vi "SoundInput-DAQ.vi"(7 "Name(\"\" to use uuid)":string="Acquisition") -> ()   [LabVIEW 2017, in "SoundInput-DAQ.lvlib"]
uses:
  SoundInput-DAQ.lvlib
  <vilib>/sound2/lvsound2.llb/Sound Data Format.ctl
  <vilib>/sound2/lvsound2.llb/Sampling Mode.ctl
  bc6f9ce3-7135-4df3-9fce-67397201bd09.vi
  f3e3012a-dc83-45d7-82c5-490bef76f43f.vi
  e2413101-be31-4c43-921b-7e7496268bc5.vi
  07cbb487-6694-43fd-ac53-f2be3466fcff.vi
  fecb174d-6823-407c-a974-ffebb4610b14.vi
  0bf643a1-791c-4b4c-b91f-da80b9c7e2fb.vi
  041ba748-83ae-40d3-86c4-8e2f4b565384.vi
  <userlib>/_NEVSTOP/Communicable State Machine(CSM)/AdvanceAPI/CSM - Revert Arguments-Safe String.vi
  <userlib>/_NEVSTOP/Communicable State Machine(CSM)/_Shared/Trim Single-line Text.vi
  <userlib>/_NEVSTOP/Communicable State Machine(CSM)/AdvanceAPI/CSM - Make String Arguments Safe.vi
  <userlib>/_NEVSTOP/Communicable State Machine(CSM)/AdvanceAPI/CSM - Break Down Multiple States String.vi
  <userlib>/_NEVSTOP/Communicable State Machine(CSM)/AdvanceAPI/CSM - Compact Multiple States.vi
  f3e3012a-dc83-45d7-82c5-490bef76f43f.vi/99de0c97-112a-4c86-9094-c187659127e1.vi
  <userlib>/_NEVSTOP/Communicable State Machine(CSM)/Utility/Build Error Cluster.vi
  0bf643a1-791c-4b4c-b91f-da80b9c7e2fb.vi/99de0c97-112a-4c86-9094-c187659127e1.vi
  <userlib>/_NEVSTOP/Communicable State Machine(CSM)/AdvanceAPI/CSM - Keywords.vi
  <vilib>/Utility/Data Type/Get Type Information.vi
  <userlib>/_NEVSTOP/Communicable State Machine(CSM)/addons/API-String-Arugments-Support/_Support/Data To SingleElementsArray_csm.vi
  <userlib>/_NEVSTOP/Communicable State Machine(CSM)/addons/API-String-Arugments-Support/_Support/Data To API String Arguments.vi
  <userlib>/_NEVSTOP/Communicable State Machine(CSM)/addons/INI-Static-Variable-Support/_Support/Parse Used Session and Name.vi
  <userlib>/_NEVSTOP/Communicable State Machine(CSM)/addons/INI-Static-Variable-Support/_Support/INI-FGV(lvlibp).vi
  <userlib>/_NEVSTOP/Communicable State Machine(CSM)/addons/INI-Static-Variable-Support/_Support/Populate String with INI Variable.vi
  <userlib>/_NEVSTOP/Communicable State Machine(CSM)/addons/API-String-Arugments-Support/_Support/Convert API String Arguments to Data(variant).vi
  <userlib>/_NEVSTOP/Communicable State Machine(CSM)/addons/API-String-Arugments-Support/_Support/SingleElementsArray To Data_csm.vi
  <userlib>/_NEVSTOP/Communicable State Machine(CSM)/addons/API-String-Arugments-Support/_Support/Query Data as API String Arguments(variant).vi
  <vilib>/sound2/lvsound2.llb/Sound Input Read (DBL).vi
  <userlib>/_NEVSTOP/Communicable State Machine(CSM)/addons/MassData-Parameter/_support/FGV-MassData(lvlibp).vi
  <userlib>/_NEVSTOP/Communicable State Machine(CSM)/_Polymophic/Add State(s) to Queue By BOOL(Element).vi
  <userlib>/_NEVSTOP/Communicable State Machine(CSM)/_Polymophic/CSM - Filter Duplicated Lines.vi
  <userlib>/_NEVSTOP/Communicable State Machine(CSM)/_Polymophic/CSM - Replace Marks in Messages.vi
  <userlib>/_NEVSTOP/Communicable State Machine(CSM)/Communicable State Machine.lvlib
  <userlib>/_NEVSTOP/Communicable State Machine(CSM)/addons/Loop-Support/CSM Loop Support.lvlib
  <userlib>/_NEVSTOP/Communicable State Machine(CSM)/_Shared/CSM Shared.lvlib
panel:
  in  "Sound Format":T1={"sample rate (S/s)"=20000.0, "number of channels"=2, "bits per sample"=16}
  in  "Device ID":u32 format="%.0x"
  in  "SamplePeroid(ms)":i32=200
  out "Raw Data":waveform(dbl)[](graph)
  in  "Cancel Button":bool
  in  "OK Button":bool
  out "Error Occurred":errorcluster
  out "State History":string
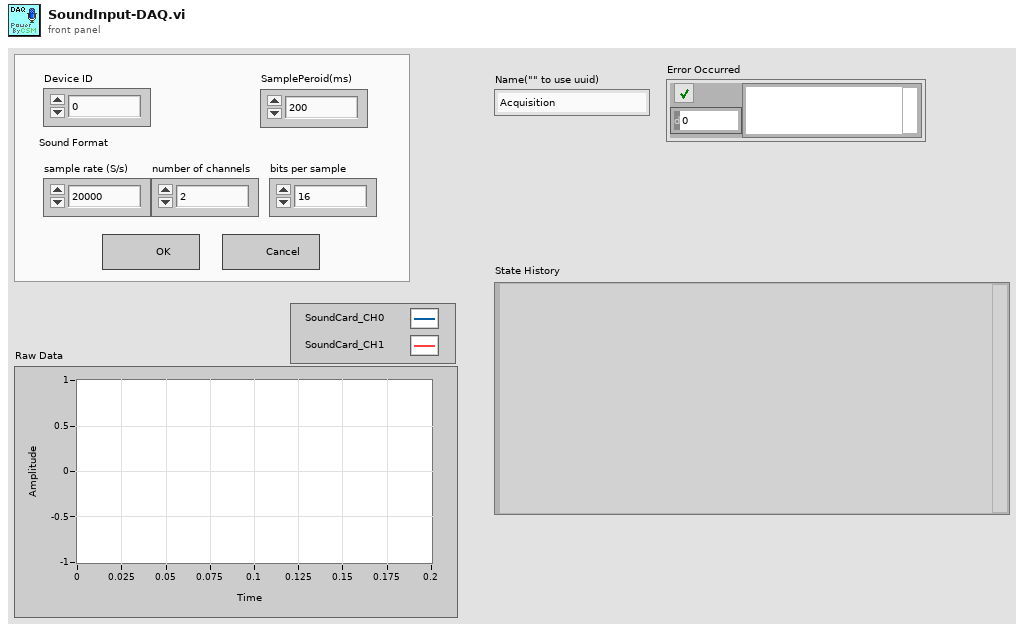
[diagram p1: front panel]
types:
  T1 = cluster{"sample rate (S/s)":dbl, "number of channels":i32, "bits per sample":i32}
  T2 = enum32{"Invalid", "Default", "Floating", "Floating/Auto-Hide", "Modal"}
  T3 = cluster{"Device ID":u32, "SamplePeroid(ms)":i32, "Sound Format":cluster{"sample rate (S/s)":dbl, "number of channels":i32, "bits per sample":i32}}
  T4 = enum32{"Invalid", "Standard", "Closed", "Hidden", "Minimized", "Maximized"}
  T5 = enum32{"invalid app kind", "Development System", "Run Time System", "Student Edition", "Embedded LabVIEW", "Evaluation", "Custom"}
  T6 = typedef "Communicable State Machine.lvlib/_CSM_Response Source Message.ctl" = cluster{"‘State":string, "’Arguments":string, "’Error":errorcluster}
  T7 = cluster{"Current VI Reference":refnum<vi>, "Close Panel on Exit?":bool}
  T8 = typedef "Sound Data Format.ctl" = cluster{"sample rate (S/s)":dbl, "number of channels":i32, "bits per sample":i32}
  T9 = cluster{"Core":cluster{"Current VI Reference":refnum<vi>, "Close Panel on Exit?":bool}, "Configuration":cluster{"Device ID":u32, "SamplePeroid(ms)":i32, "Sound Format":T8}, "State":enum16{"Idle", "Acquiring"}, "Number of Samples/ch":i32, "timestamp":timestamp}
  T10 = cluster{"Device ID":u32, "SamplePeroid(ms)":i32, "Sound Format":T8}
  T11 = typedef "Sampling Mode.ctl" = i32
  T12 = typedef "Sound Input Task ID.ctl" = u32
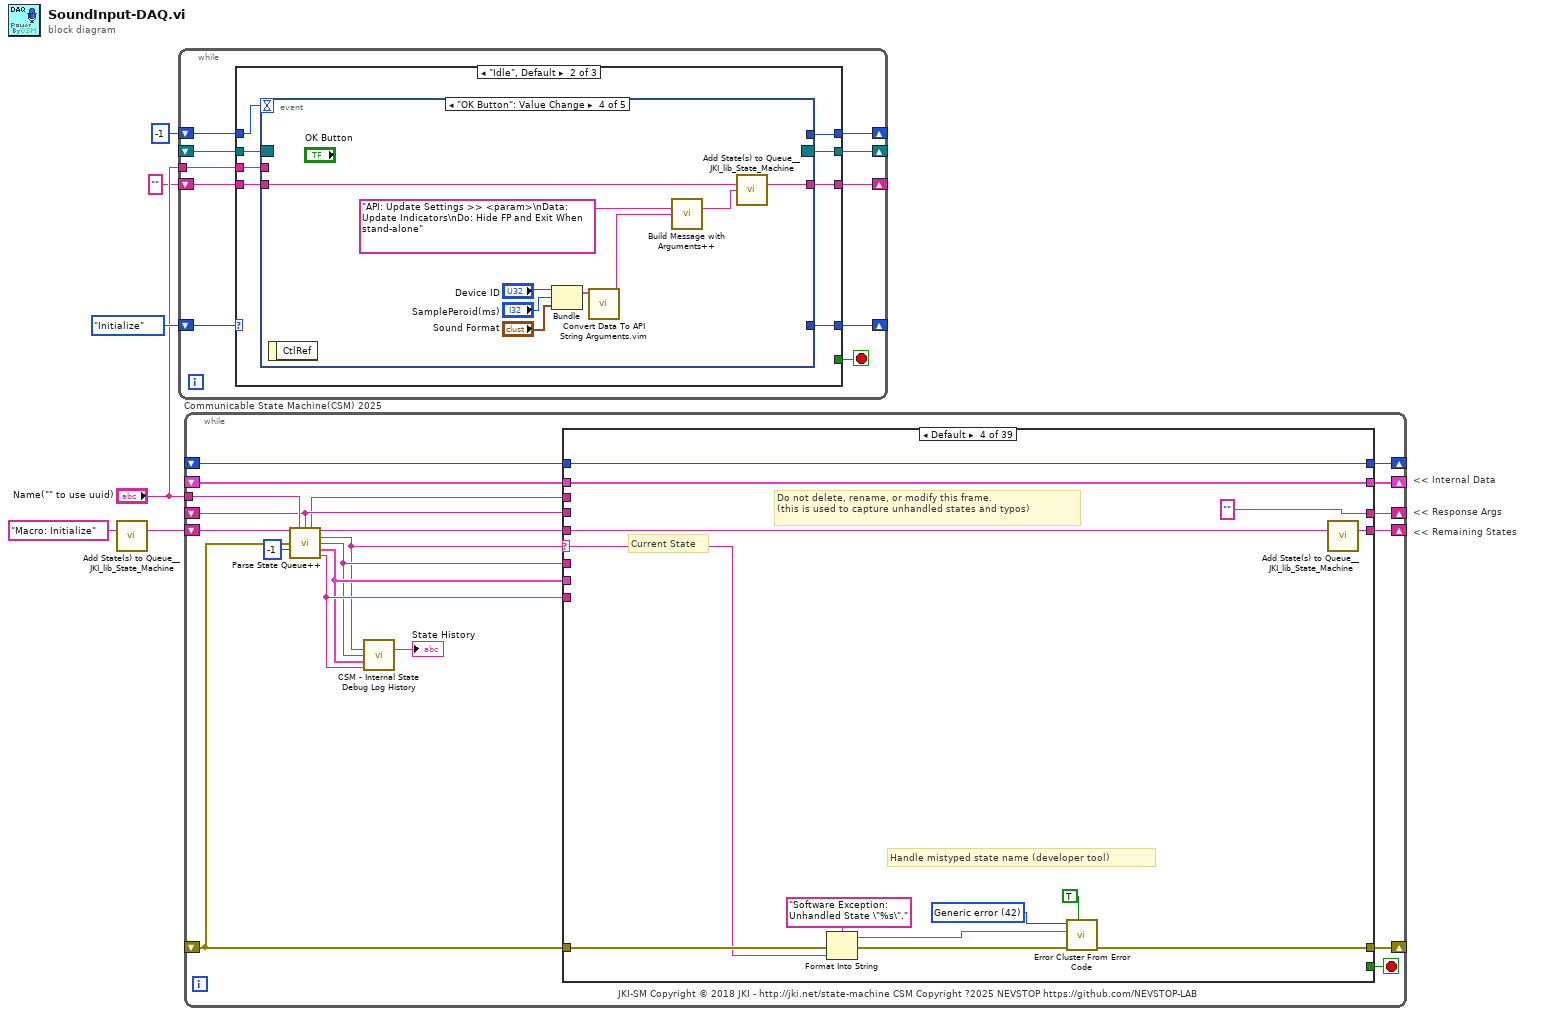
[diagram p0: block diagram]
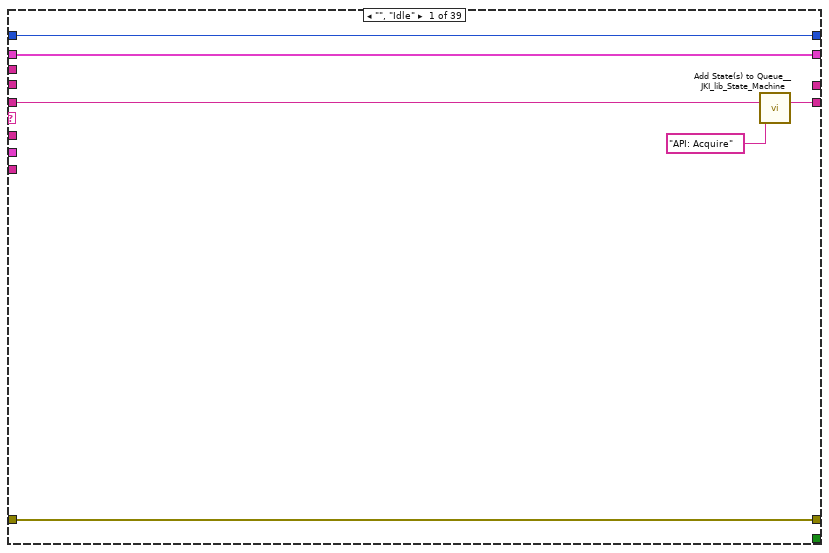
[diagram p2: hidden frame]
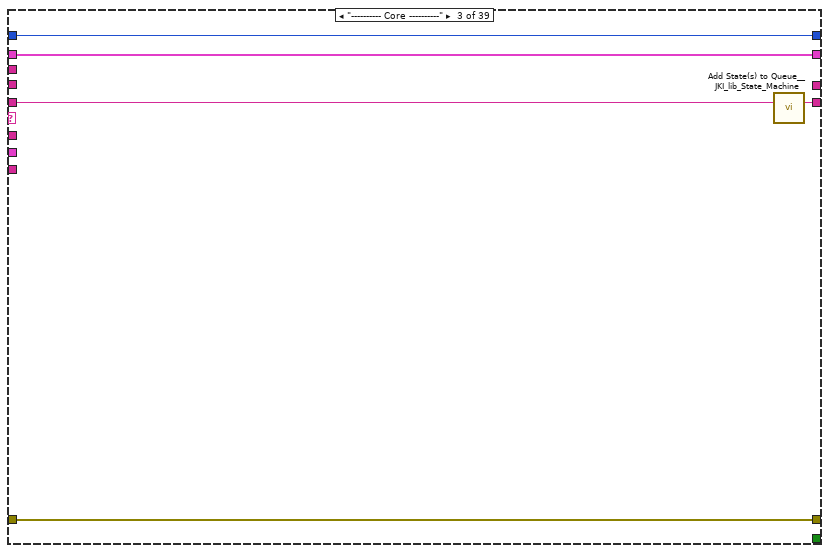
[diagram p4: hidden frame]
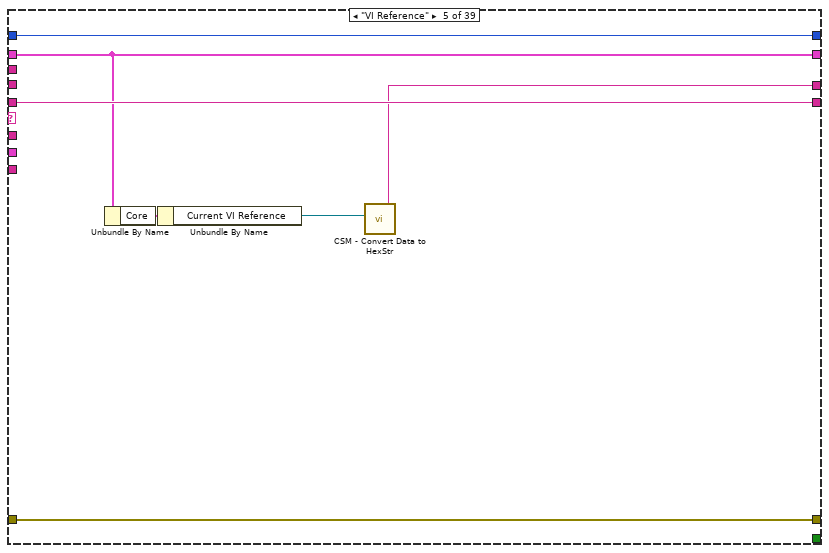
[diagram p5: hidden frame]
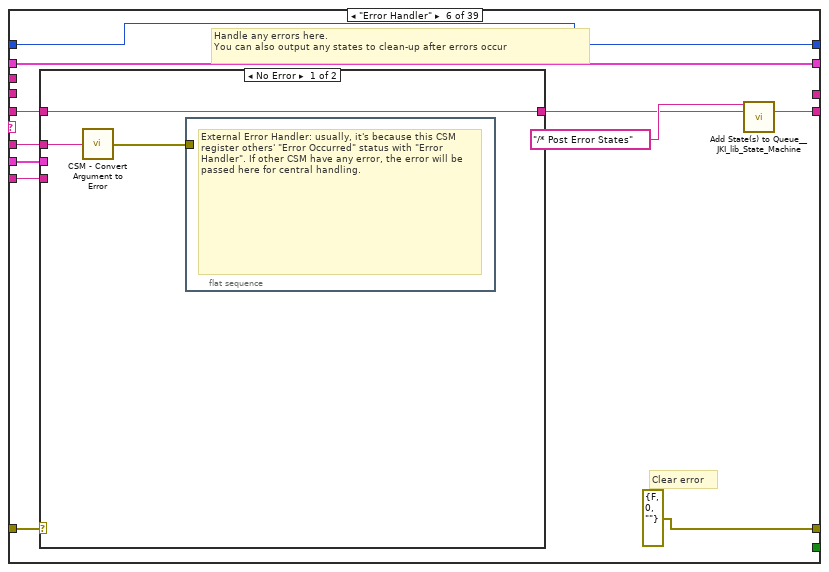
[diagram p6: hidden frame]
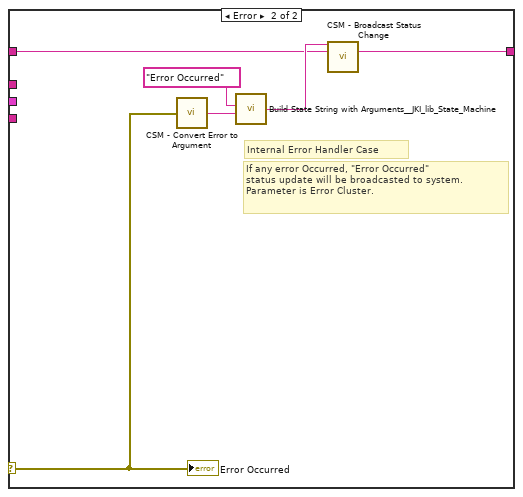
[diagram p7: hidden frame]
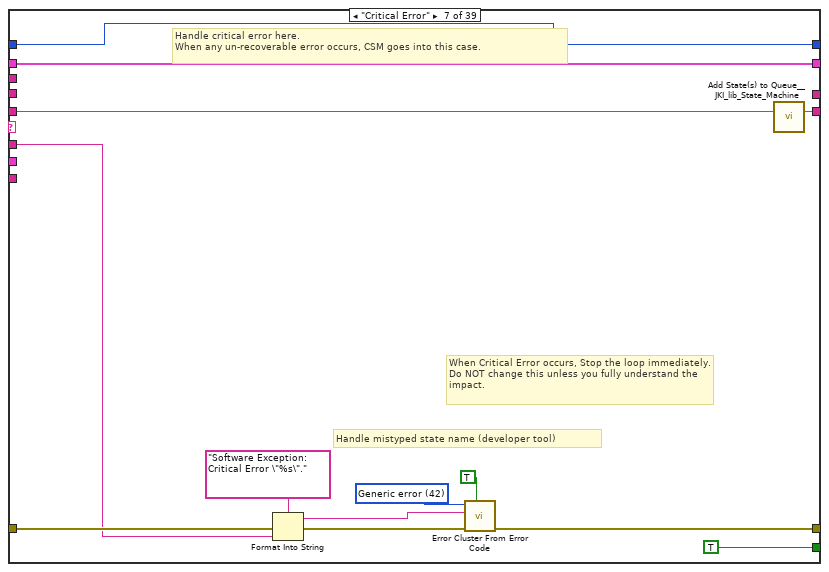
[diagram p8: hidden frame]
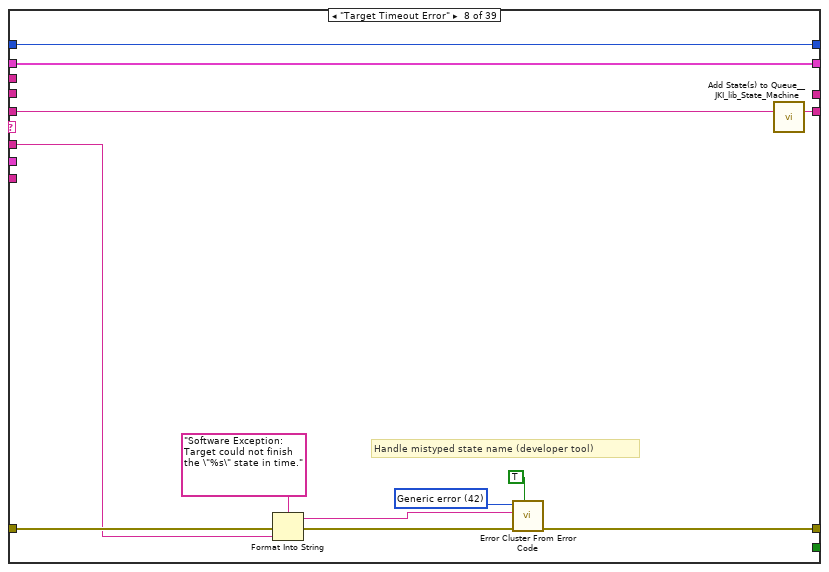
[diagram p9: hidden frame]
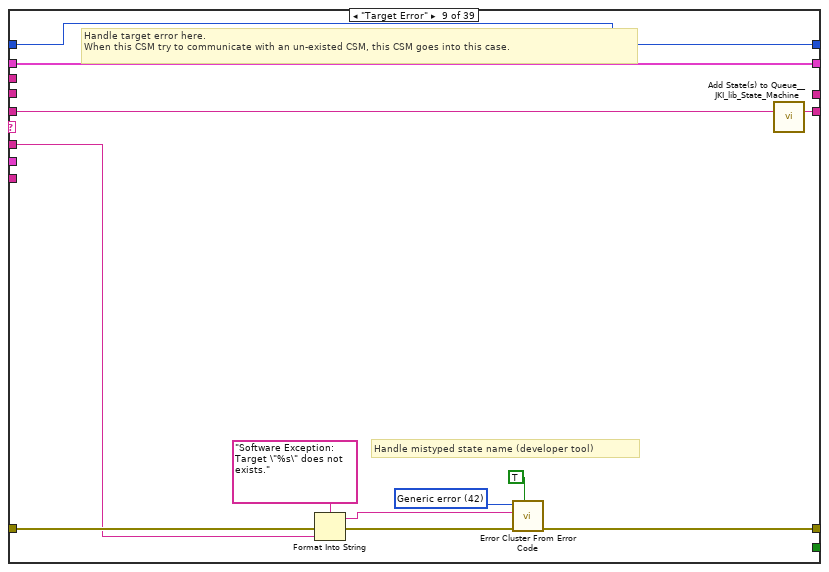
[diagram p10: hidden frame]
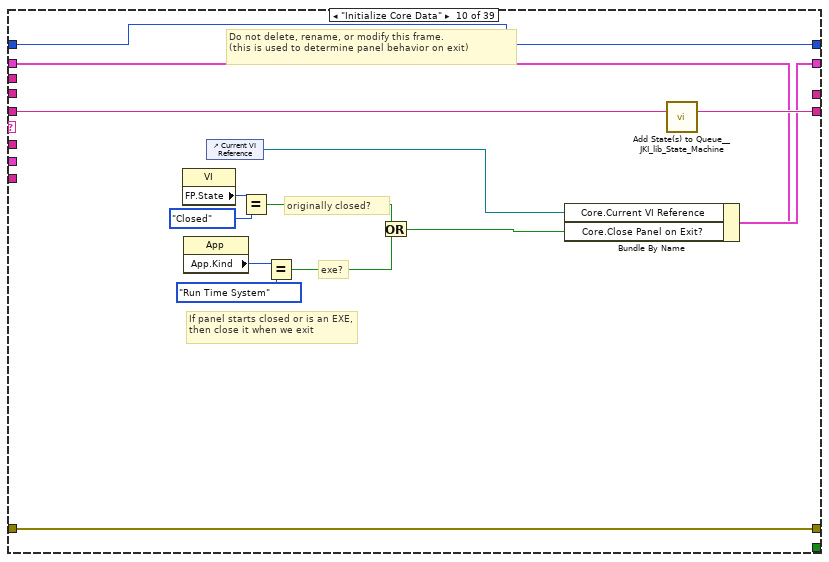
[diagram p11: hidden frame]
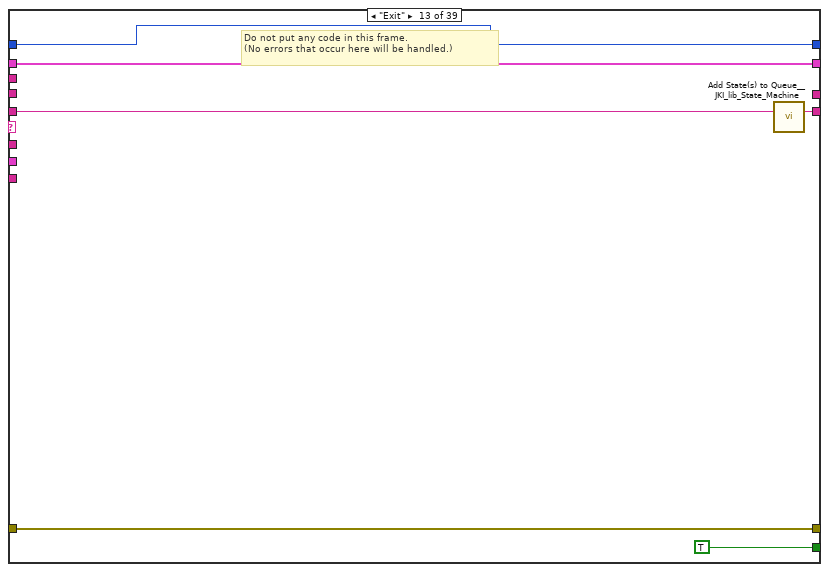
[diagram p14: hidden frame]
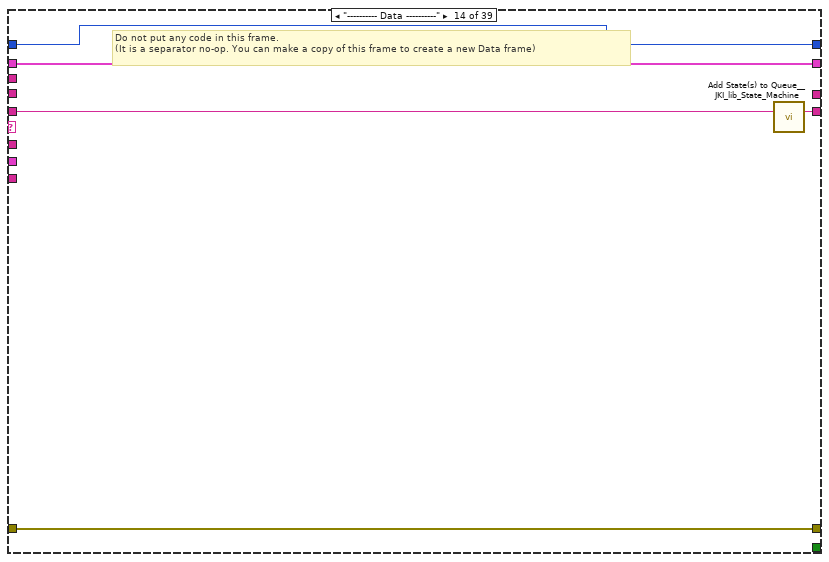
[diagram p15: hidden frame]
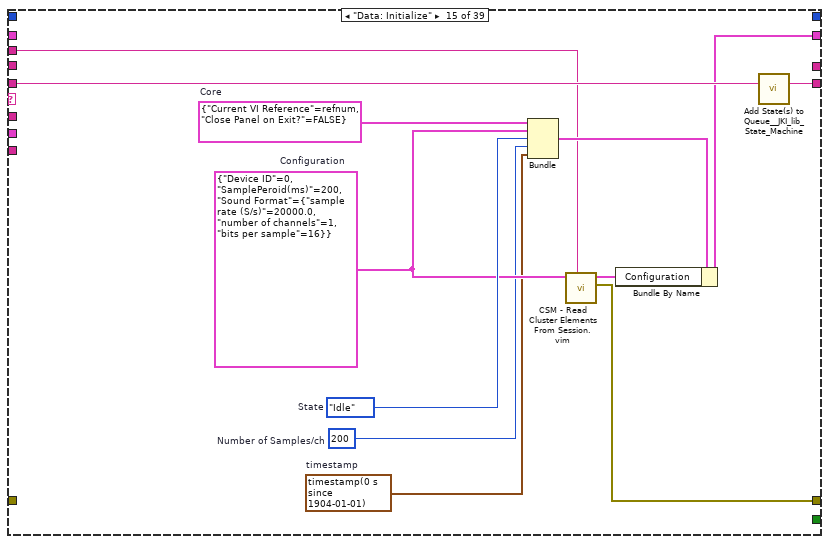
[diagram p16: hidden frame]
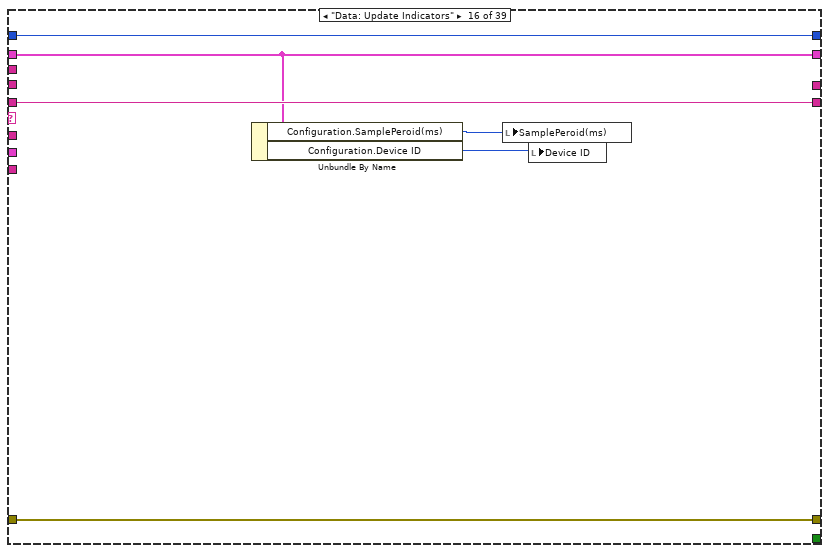
[diagram p17: hidden frame]
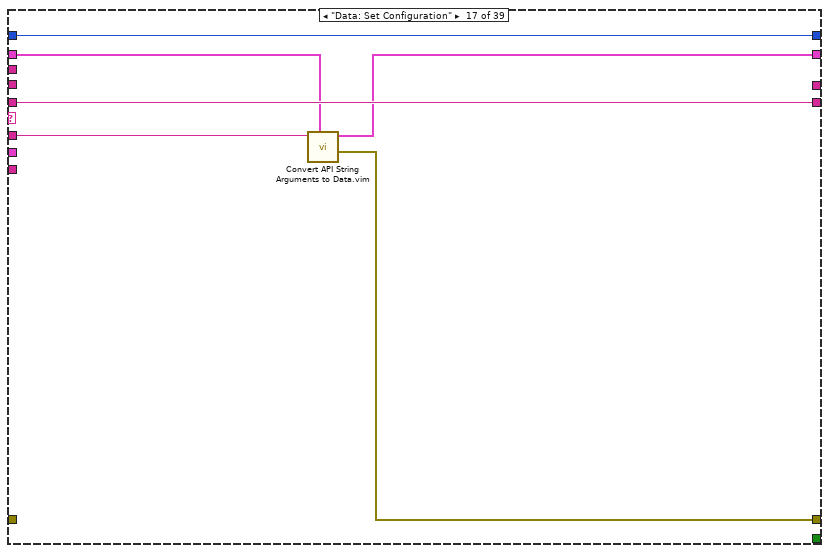
[diagram p18: hidden frame]
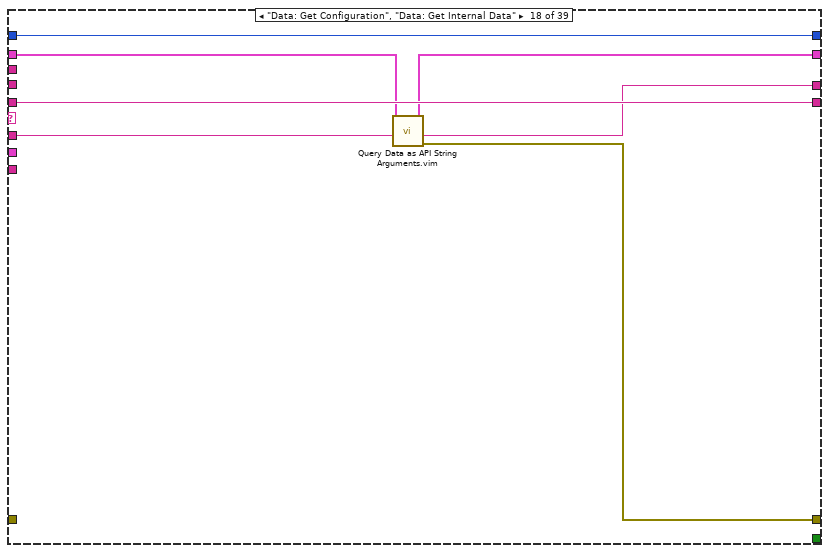
[diagram p19: hidden frame]
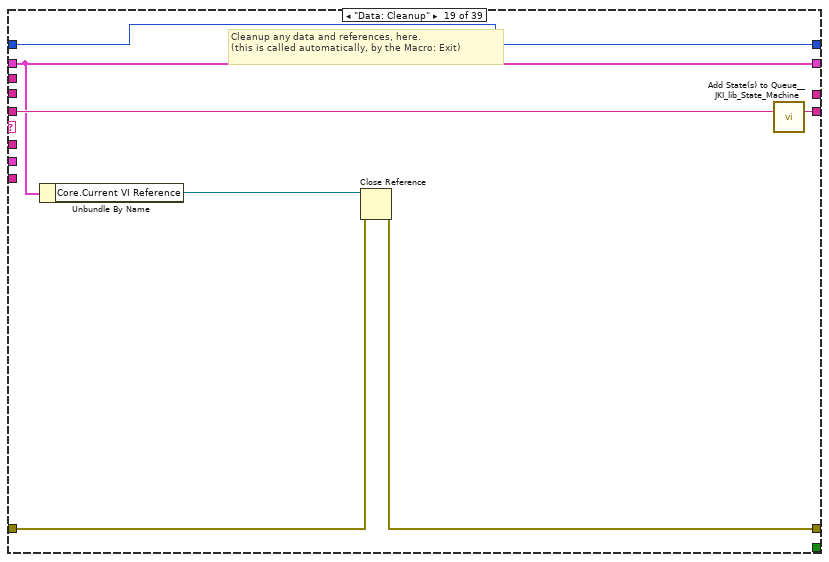
[diagram p20: hidden frame]
diagram:
  # "<< Internal Data"
  # "<< Response Args"
  # "<< Remaining States"
  n1 = call <vilib>:"Add State(s) to Queue__JKI_lib_State_Machine.vi"("State(s) in (\"\")"="Macro: Initialize") -> ("States Out"=w5:string)  [unwired: 14 in]
  n2 = while {
    shift-right: [w12] -> _
    shift-left: enum16{"Idle", "Initialize", "Exit"}."Initialize" -> [w16]
    tunnel: "Name(\"\" to use uuid)" -> [w15]
    shift-right: [w14] -> _
    shift-left: _ -> [w13]
    shift-right: [w9] -> _
    shift-left: "" -> [w10]
    shift-right: [w7] -> _
    shift-left: -1 -> [w8]
    stop <- w11 stop-if-true
    n3 = case shown="\"Idle\", Default" w16 {
      tunnel: w15 -> [w24 w27 _]
      tunnel: [w21 w32 _] -> w14
      tunnel: w13 -> [_ w31 w61]
      tunnel: [enum16{"Idle", "Initialize", "Exit"}."Idle" w30 _] -> w12
      tunnel: [_ _ TRUE] -> w11
      tunnel: w10 -> [w19 w29 w58]
      tunnel: [w19 w28 w58] -> w9
      tunnel: w8 -> [w18 w25 w57]
      tunnel: [w18 w26 w57] -> w7
      frame "Initialize" {
        n4 = call <userlib>:"CSM - Module Exit Event.vi"("Name (\"\" to Use UUID) In"=w24) -> ("error out"=w23:errorcluster, "CSM Exit Event"=w22:refnum<user-event>)  [unwired: 8 in, 1 out]
        n5 = register-events(error in=w23, w22) -> (reference out=w21:refnum<event-registration>)  [unwired: 1 in, 1 out]
        n6 = property class="VI"("FP.Behavior"=T2."Default" ("Front Panel Window:Behavior")) -> ()  [unwired: 2 in, 2 out]
      }
      frame "Idle", Default {
        n7 = event shown="[3] \"OK Button\": Value Change" {
          selector: w31 -> [_ _ _ _ _]
          dyn-events: [_ _ _ _ _] -> w32
          timeout: w25 -> [_ _ _ _ _]
          tunnel: [_ _ enum16{"Idle", "Initialize", "Exit"}."Exit" _ _] -> w30
          tunnel: w29 -> [w36 w40 w42 w52 w55]
          tunnel: [w37 w39 w42 w45 w54] -> w28
          tunnel: w27 -> [w34 _ _ _ _]
          tunnel: [-1 _ _ _ _] -> w26
          event Timeout {
            n8 = event-data() -> ()  [unwired: 1 in, 1 out]
            n9 = call-poly <userlib>:"CSM - Filter JKISM String Queue.vi"("States In"=w36) -> ("States Out"=w33:string)  [unwired: 14 in]
            n10 = call <userlib>:"CSM - Forward UI Operations to CSM.vi"("Name (\"\" to Use UUID)"=w34, "State(s) In (\"\")"=w33) -> ("States Out"=w37:string)  [unwired: 8 in, 1 out]
          }
          event Panel Close? {
            n11 = event-data() -> ()  [unwired: 1 in, 2 out]
            n12 = call <vilib>:"Add State(s) to Queue__JKI_lib_State_Machine.vi"("State(s) in (\"\")"=w40, "State(s) at Back (\"\")"="Do: Hide FP and Exit When stand-alone" ("State(s) at Back (\"\")")) -> ("States Out"=w39:string)  [unwired: 13 in]
            n13 = event-data("Discard?"=TRUE) -> ()  [unwired: 1 in, 1 out]
          }
          event User Event {
            n14 = event-data() -> ()  [unwired: 1 in, 1 out]
          }
          event "OK Button": Value Change {
            n15 = event-data() -> ()  [unwired: 1 in, 1 out]
            n16 = Bundle("Device ID"="Device ID", "SamplePeroid(ms)"="SamplePeroid(ms)", "Sound Format"="Sound Format") -> (w47:T3)  [unwired: 1 in]
            n17 = call "Convert Data To API String Arguments.vim"("Data"=w47) -> ("API String"=w50:string)  [unwired: 7 in, 1 out]
            n18 = call-poly <userlib>:"Build Message with Arguments++.vi"("States With Replace Token"="API: Update Settings >> <param>\nData: Update Indicators\nDo: Hide FP and Exit When stand-alone" ("State"), "<param>"=w50) -> ("States"=w44:string)  [unwired: 13 in]
            n19 = call <vilib>:"Add State(s) to Queue__JKI_lib_State_Machine.vi"("State(s) in (\"\")"=w52, "State(s) at Back (\"\")"=w44) -> ("States Out"=w45:string)  [unwired: 13 in]
          }
          event "Cancel Button": Value Change {
            n20 = event-data() -> ()  [unwired: 1 in, 1 out]
            n21 = call <vilib>:"Add State(s) to Queue__JKI_lib_State_Machine.vi"("State(s) in (\"\")"=w55, "State(s) at Back (\"\")"="Do: Hide FP and Exit When stand-alone" ("State(s) at Back (\"\")")) -> ("States Out"=w54:string)  [unwired: 13 in]
          }
        }
      }
      frame "Exit" {
        n22 = Unregister For Events(event registration refnum=w61) -> (error out=w60:errorcluster)  [unwired: 1 in]
        n23 = call <vilib>:"Clear Errors.vi"("error in (no error)"=w60) -> ()  [unwired: 5 in, 2 out]
        n24 = property class="VI"("FP.Behavior"=T2."Default" ("Front Panel Window:Behavior")) -> ()  [unwired: 2 in, 2 out]
      }
    }
  }
  n25 = while "Communicable State Machine(CSM) 2025" {
    shift-right: [w76] -> _
    shift-left: _ -> [w66]
    shift-right: [w79] -> _
    shift-left: _ -> [w75]
    shift-right: [w78] -> _
    shift-left: w5 -> [w80]
    tunnel: "Name(\"\" to use uuid)" -> [w73]
    shift-right: [w74] -> _
    shift-left: _ -> [w68]
    shift-right: [w63] -> _
    shift-left: _ -> [w62]
    stop <- w77 stop-if-true
    # "JKI-SM Copyright © 2018 JKI - http://jki.net/state-machine CSM Copyright ?2025 NEVSTOP https://github.com/NEVSTOP-LAB"
    n26 = call <userlib>:"Parse State Queue++.vi"("State Queue"=w80, "Name (\"\" to Use UUID)"=w73, "Response Arguments"=w68, "Previous Error"=w75, "Dequeue (1 ms)"=-1 ("Dequeue Timeout(1ms)")) -> ("Name Used"=w67:string, "Remaining States"=w81:string, "Current State"=w69:string, "Arguments"=w70:string, "Additional Information"=w71:T6, "Source CSM"=w72:string)  [unwired: 5 in]
    n27 = call <userlib>:"CSM - Internal State Debug Log History.vi"("State"=w69, "Arguments (\"\")"=w70, ">> Response Source Message >>"=w71, "Source (\"\")"=w72) -> ("Debug Log"=→"State History":string)  [unwired: 11 in]
    n28 = case shown="Default" w69 {
      selector: w69 -> [_ _ _ w99 _ _ _ _ _ _ _ _ _ _ _ _ _ _ _ _ _ _ _ _ _ _ _ _ _ _ _ _ _ _ w386 _ _ _ _]
      tunnel: w81 -> [w84 w90 w96 w103 w115 w121 w143 w156 w168 w187 w190 w194 w201 w206 w218 w223 w230 w237 w244 w249 w255 w261 w264 w269 w283 w297 w309 w323 w326 w331 w340 w373 w378 w381 w389 w398 w403 w411 w482]
      tunnel: w70 -> [_ _ _ _ _ w120 w139 w152 w164 _ _ _ _ _ _ _ w228 w234 _ _ _ _ _ _ _ w293 _ _ _ _ _ _ _ _ w385 _ _ w408 _]
      tunnel: w66 -> [w86 w89 w93 w101 w114 w126 w141 w154 w166 w180 w189 w193 w199 w203 _ w221 w229 w236 w239 w246 w252 w258 w263 w272 w279 w295 w308 w322 w324 w330 w342 w372 w377 w380 w387 w399 w402 w410 w487]
      tunnel: [w87 w91 w94 w105 w116 errorcluster {"status"=FALSE, "code"=0, "source"=""} ("error out") w145 w151 w163 w184 w191 w195 w198 w204 w209 w224 w226 w232 w240 w247 w253 w259 w265 w270 w281 w289 w310 w319 _ w332 w344 _ w374 w382 w390 w400 w404 w407 w488] -> w79
      tunnel: w75 -> [w87 w91 w94 w104 w116 w124 w144 w157 w169 w184 w191 w195 w198 w204 _ w224 _ _ w241 w247 w253 w259 w265 w270 w281 _ w310 _ _ w332 w345 _ _ w382 w390 w400 w404 w409 w488]
      tunnel: [w85 w90 w95 w102 w115 w122 w142 w155 w167 w186 w190 w194 w200 w205 w217 w223 w230 w237 w243 w248 w254 w260 w264 w268 w282 w297 w309 w323 w326 w331 w341 w373 w378 w381 w388 w397 w403 w411 w483] -> w78
      tunnel: [_ _ _ _ _ _ TRUE _ _ _ _ _ TRUE _ _ _ _ _ _ _ _ _ _ _ _ _ _ _ _ _ _ _ _ _ _ _ _ _ _] -> w77
      tunnel: [w86 w89 w93 w101 w114 w126 w141 w154 w166 w185 w189 w193 w199 w203 w211 w221 w227 w235 w239 w246 w252 w258 w263 w271 w279 w296 w308 w312 w324 w328 w343 w371 w377 w380 w383 w399 w402 w410 w487] -> w76
      tunnel: w72 -> [_ _ _ _ _ w119 _ _ _ _ _ _ _ _ _ _ _ _ _ _ _ _ _ _ _ _ _ _ _ _ _ _ _ _ _ _ _ _ _]
      tunnel: w71 -> [_ _ _ _ _ w118 _ _ _ _ _ _ _ _ _ _ _ _ _ _ _ _ _ _ _ _ _ _ _ _ _ _ _ _ _ _ _ _ _]
      tunnel: [_ _ _ "" w111 _ _ _ _ _ _ _ _ _ _ _ _ w233 _ _ _ _ _ _ _ _ _ _ _ _ w338 _ _ _ _ _ _ _ _] -> w74
      tunnel: w67 -> [_ _ _ _ _ _ _ _ _ _ _ _ _ _ w213 _ _ _ _ _ _ _ _ _ _ w288 _ _ _ _ _ _ _ _ _ _ _ _ _]
      tunnel: w68 -> [_ _ _ _ _ _ _ _ _ _ _ _ _ _ _ _ _ _ _ _ _ _ _ _ _ _ _ _ _ _ _ _ _ _ _ _ _ _ _]
      tunnel: [w82 w88 w92 w97 w110 w117 w137 w150 w162 w174 w188 w192 w196 w202 _ w220 w225 w231 w238 w245 w250 w256 w262 w266 w278 w286 w307 w318 w325 w329 w335 w369 _ w379 w384 w396 w401 w405 w486] -> w63
      tunnel: w62 -> [w82 w88 w92 w97 w110 w117 w137 w150 w162 w174 w188 w192 w196 w202 _ w220 w225 w231 w238 w245 w250 w256 w262 w266 w278 w286 w307 _ w325 w329 w336 w369 w376 w379 w384 w396 w401 w405 w486]
      frame "", "Idle" {
        n29 = call <vilib>:"Add State(s) to Queue__JKI_lib_State_Machine.vi"("State(s) in (\"\")"=w84, "State(s) at Back (\"\")"="API: Acquire" ("State(s) in Front (\"\")")) -> ("States Out"=w85:string)  [unwired: 13 in]
      }
      frame "CSM Documentation" {
        # "CSM Documentation"
        # "State Syntax:\nStateCategory: State >> Argument -@ CSMName\nStateCategory: State >> Argument -> CSMName\n\nLine Terminator: Line feed"
        # "Commenting:\nTo add a comment use \"//\" or \"#\" and all text to the right will be ignored\nCommenting Example:\nUI: Initialize // This initializes the UI\n// Another comment line"
        # "Example:\nUI: Help >> About -@Main\nUI: Help >> About ->Main\n\nWhere \"UI\" is the state category\nWhere \"Help\" is the state\nWhere \"About\" is the argument\nWhere \"Main\" is the Name of CSM,which actually run the \"UI: Help >> About\"\n\n    \"-@\" stands for sync state. Current CSM will wait until the state is finished. \n            - if \"Main\" named CSM does not exist, \"Target Error\" will occur.\n            - if \"Main\" named CSM is in another sync remote state, \"Target Busy Error\" will occur.\n            - if \"Main\" named CSM could not finish the state in time, \"Target Timeout Error\" will occur.\n            - if everything is right. \"Response\" will occur with Argument back from \"Main\" named CSM. \n\n    \"->\" stands for async state. Current CSM will post the state and continue to next state in next iteration.\n            - if \"Main\" named CSM does not exist, \"Target Error\" will occur.\n            - if everything is right. \"Async Message Posted\" will occur.\n            - After State is finished. Caller will receive a \"Async Response\" state from callee.\n\nWhen duplicated name is used for multiple CSM module or some framework problem happens, \"Critical Error\" will occur."
      }
      frame "---------- Core ----------" {
        n30 = call <vilib>:"Add State(s) to Queue__JKI_lib_State_Machine.vi"("State(s) in (\"\")"=w96) -> ("States Out"=w95:string)  [unwired: 14 in]
      }
      frame Default {
        w108 = 42 items=["No error", "Argument error", "Memory is full", "Out of zone", "End of file", "File already open", "Generic file I/O error", "File not found", "File permission error", "Disk is full", "Duplicate path", "Too many files open", "System feature not enabled", "Resource file not found", "Cannot add resource", "Resource not found", "Image not found", "Image memory error", "Pen does not exist", "Config type invalid", "Config token not found", "Config parse error", "Config memory error", "Bad external code format", "Bad external code offset", "External code not present", "Null window", "Destroy window error", "Null menu", "Print aborted", "Bad print record", "Print driver error", "Windows error during printing", "Memory error during printing", "Print dialog error", "Generic print error", "Invalid device refnum", "Device not found", "Device parameter error", "Device unit error", "Cannot open device", "Device call aborted", "Generic error", "Cancelled by user", "Object ID too low", "Object ID too high", "Object not in heap", "Unknown heap", "Unknown object (invalid DefProc)", "Unknown object (DefProc not in table)", "Message out of range", "Invalid (null) method", "Unknown message", "Manager call not supported", "Bad address", "Network operation in progress", "Network operation timed out", "Connection is busy", "Network attribute not supported", "Network error", "Address in use", "System out of memory", "Connection aborted", "Connection refused", "Not connected", "Already connected", "Connection closed", "Initialization error (interapplication manager)", "Bad occurrence", "Wait on unbound occurrence handler", "Occurrence queue overflow", "Datalog type conflict", "Unused", "Unrecognized type (interapplication manager)", "Memory corrupt", "Failed to make temporary DLL", "Old CIN version", "Drag socket not found", "Failed to load drop-object", "Failed to register OLE object", "Failed to release OLE object", "Format specifier type mismatch", "Unknown format specifier", "Too few format specifiers", "Too many format specifiers", "Scan failed", "Newer CIN version", "Error converting to variant", "Runtime menu error", "Password tampered", "Variant attribute not found", "Incompatible variant data type", "Event data is not available", "Event Store is not present", "Occurrence is not found", "Event Queue is not created", "Event info is not available", "Refnum passed is NULL", "Error retrieving Class GUID", "Error retrieving CoClass GUID", "Error retrieving TypeLib GUID.", "Bad built application magic bytes.", "Specific driver is different from the specific driver associated with the Logical Name.", "There is no session opened to the class driver.", "Max Error", "MAX - Error with config objects", "MAX - Error loading configuration", "MAX - Group not supported"]
        # "Current State"
        # "Do not delete, rename, or modify this frame.\n(this is used to capture unhandled states and typos)"
        # "Handle mistyped state name (developer tool)"
        n31 = Format Into String(format string="Software Exception: Unhandled State \"%s\"." ("message"), error in=w104, w99) -> (resulting string=w107:string, error out=w106:errorcluster)  [unwired: 1 in]
        n32 = call <vilib>:"Error Cluster From Error Code.vi"("show call chain? (False)"=TRUE, "error in (no error)"=w106, "error message (\"\")"=w107, "error code (0)"=w108) -> ("error out"=w105:errorcluster)  [unwired: 5 in]
        n33 = call <vilib>:"Add State(s) to Queue__JKI_lib_State_Machine.vi"("State(s) in (\"\")"=w103) -> ("States Out"=w102:string)  [unwired: 14 in]
      }
      frame "VI Reference" {
        n34 = Unbundle By Name(w114) -> ("Core"=w113:T7)
        n35 = Unbundle By Name(w113) -> ("Current VI Reference"=w112:refnum<vi>)
        n36 = call <userlib>:"CSM - Convert Data to HexStr.vi"("Variant"=w112) -> ("HEX String (0-9,A-F)"=w111:string)  [unwired: 8 in]
      }
      frame "Error Handler" {
        # "Handle any errors here.\nYou can also output any states to clean-up after errors occur"
        # "Clear error"
        n37 = case shown="No Error" w124 {
          selector: w124 -> [_ w131]
          tunnel: [w130 w133] -> w123
          tunnel: w121 -> [w130 w132]
          tunnel: w120 -> [w129 _]
          tunnel: w119 -> [_ _]
          tunnel: w118 -> [_ _]
          frame No Error {
            n38 = call <userlib>:"CSM - Convert Argument to Error.vi"("Argument"=w129) -> ("Error"=w128:errorcluster)  [unwired: 4 in]
            n39 = flat-sequence {
              tunnel: w128 -> [_]
              frame #0 {
                # "External Error Handler: usually, it's because this CSM register others' \"Error Occurred\" status with \"Error Handler\". If other CSM have any error, the error will be passed here for central handling."
              }
            }
          }
          frame Error {
            # "Internal Error Handler Case"
            # "If any error Occurred, \"Error Occurred\" \nstatus update will be broadcasted to system.\nParameter is Error Cluster."
            n40 = call <userlib>:"CSM - Convert Error to Argument.vi"("Error"=w131) -> ("Argument"=w135:string)  [unwired: 4 in]
            n41 = call <vilib>:"Build State String with Arguments__JKI_lib_State_Machine.vi"("Arguments (\"\")"=w135, "State"="Error Occurred" ("Status with Arguments")) -> ("State with Arguments"=w134:string)  [unwired: 4 in]
            n42 = call <userlib>:"CSM - Broadcast Status Change.vi"("Status With Arguments"=w134, "State Queue"=w132) -> ("Remaining States"=w133:string)  [unwired: 13 in]
            "Error Occurred" <- w131
          }
        }
        n43 = call <vilib>:"Add State(s) to Queue__JKI_lib_State_Machine.vi"("State(s) in Front (\"\")"="/* Post Error States", "State(s) in (\"\")"=w123) -> ("States Out"=w122:string)  [unwired: 13 in]
      }
      frame "Critical Error" {
        w148 = 42 items=["No error", "Argument error", "Memory is full", "Out of zone", "End of file", "File already open", "Generic file I/O error", "File not found", "File permission error", "Disk is full", "Duplicate path", "Too many files open", "System feature not enabled", "Resource file not found", "Cannot add resource", "Resource not found", "Image not found", "Image memory error", "Pen does not exist", "Config type invalid", "Config token not found", "Config parse error", "Config memory error", "Bad external code format", "Bad external code offset", "External code not present", "Null window", "Destroy window error", "Null menu", "Print aborted", "Bad print record", "Print driver error", "Windows error during printing", "Memory error during printing", "Print dialog error", "Generic print error", "Invalid device refnum", "Device not found", "Device parameter error", "Device unit error", "Cannot open device", "Device call aborted", "Generic error", "Cancelled by user", "Object ID too low", "Object ID too high", "Object not in heap", "Unknown heap", "Unknown object (invalid DefProc)", "Unknown object (DefProc not in table)", "Message out of range", "Invalid (null) method", "Unknown message", "Manager call not supported", "Bad address", "Network operation in progress", "Network operation timed out", "Connection is busy", "Network attribute not supported", "Network error", "Address in use", "System out of memory", "Connection aborted", "Connection refused", "Not connected", "Already connected", "Connection closed", "Initialization error (interapplication manager)", "Bad occurrence", "Wait on unbound occurrence handler", "Occurrence queue overflow", "Datalog type conflict", "Unused", "Unrecognized type (interapplication manager)", "Memory corrupt", "Failed to make temporary DLL", "Old CIN version", "Drag socket not found", "Failed to load drop-object", "Failed to register OLE object", "Failed to release OLE object", "Format specifier type mismatch", "Unknown format specifier", "Too few format specifiers", "Too many format specifiers", "Scan failed", "Newer CIN version", "Error converting to variant", "Runtime menu error", "Password tampered", "Variant attribute not found", "Incompatible variant data type", "Event data is not available", "Event Store is not present", "Occurrence is not found", "Event Queue is not created", "Event info is not available", "Refnum passed is NULL", "Error retrieving Class GUID", "Error retrieving CoClass GUID", "Error retrieving TypeLib GUID.", "Bad built application magic bytes.", "Specific driver is different from the specific driver associated with the Logical Name.", "There is no session opened to the class driver.", "Max Error", "MAX - Error with config objects", "MAX - Error loading configuration", "MAX - Group not supported"]
        # "Handle critical error here.\nWhen any un-recoverable error occurs, CSM goes into this case."
        # "When Critical Error occurs, Stop the loop immediately. Do NOT change this unless you fully understand the impact."
        # "Handle mistyped state name (developer tool)"
        n44 = Format Into String(format string="Software Exception: Critical Error \"%s\"." ("message"), error in=w144, w139) -> (resulting string=w147:string, error out=w146:errorcluster)  [unwired: 1 in]
        n45 = call <vilib>:"Error Cluster From Error Code.vi"("show call chain? (False)"=TRUE, "error in (no error)"=w146, "error message (\"\")"=w147, "error code (0)"=w148) -> ("error out"=w145:errorcluster)  [unwired: 5 in]
        n46 = call <vilib>:"Add State(s) to Queue__JKI_lib_State_Machine.vi"("State(s) in (\"\")"=w143) -> ("States Out"=w142:string)  [unwired: 14 in]
      }
      frame "Target Timeout Error" {
        w160 = 42 items=["No error", "Argument error", "Memory is full", "Out of zone", "End of file", "File already open", "Generic file I/O error", "File not found", "File permission error", "Disk is full", "Duplicate path", "Too many files open", "System feature not enabled", "Resource file not found", "Cannot add resource", "Resource not found", "Image not found", "Image memory error", "Pen does not exist", "Config type invalid", "Config token not found", "Config parse error", "Config memory error", "Bad external code format", "Bad external code offset", "External code not present", "Null window", "Destroy window error", "Null menu", "Print aborted", "Bad print record", "Print driver error", "Windows error during printing", "Memory error during printing", "Print dialog error", "Generic print error", "Invalid device refnum", "Device not found", "Device parameter error", "Device unit error", "Cannot open device", "Device call aborted", "Generic error", "Cancelled by user", "Object ID too low", "Object ID too high", "Object not in heap", "Unknown heap", "Unknown object (invalid DefProc)", "Unknown object (DefProc not in table)", "Message out of range", "Invalid (null) method", "Unknown message", "Manager call not supported", "Bad address", "Network operation in progress", "Network operation timed out", "Connection is busy", "Network attribute not supported", "Network error", "Address in use", "System out of memory", "Connection aborted", "Connection refused", "Not connected", "Already connected", "Connection closed", "Initialization error (interapplication manager)", "Bad occurrence", "Wait on unbound occurrence handler", "Occurrence queue overflow", "Datalog type conflict", "Unused", "Unrecognized type (interapplication manager)", "Memory corrupt", "Failed to make temporary DLL", "Old CIN version", "Drag socket not found", "Failed to load drop-object", "Failed to register OLE object", "Failed to release OLE object", "Format specifier type mismatch", "Unknown format specifier", "Too few format specifiers", "Too many format specifiers", "Scan failed", "Newer CIN version", "Error converting to variant", "Runtime menu error", "Password tampered", "Variant attribute not found", "Incompatible variant data type", "Event data is not available", "Event Store is not present", "Occurrence is not found", "Event Queue is not created", "Event info is not available", "Refnum passed is NULL", "Error retrieving Class GUID", "Error retrieving CoClass GUID", "Error retrieving TypeLib GUID.", "Bad built application magic bytes.", "Specific driver is different from the specific driver associated with the Logical Name.", "There is no session opened to the class driver.", "Max Error", "MAX - Error with config objects", "MAX - Error loading configuration", "MAX - Group not supported"]
        # "Handle mistyped state name (developer tool)"
        n47 = Format Into String(format string="Software Exception: Target could not finish the \"%s\" state in time." ("message"), error in=w157, w152) -> (resulting string=w159:string, error out=w158:errorcluster)  [unwired: 1 in]
        n48 = call <vilib>:"Error Cluster From Error Code.vi"("show call chain? (False)"=TRUE, "error in (no error)"=w158, "error message (\"\")"=w159, "error code (0)"=w160) -> ("error out"=w151:errorcluster)  [unwired: 5 in]
        n49 = call <vilib>:"Add State(s) to Queue__JKI_lib_State_Machine.vi"("State(s) in (\"\")"=w156) -> ("States Out"=w155:string)  [unwired: 14 in]
      }
      frame "Target Error" {
        w172 = 42 items=["No error", "Argument error", "Memory is full", "Out of zone", "End of file", "File already open", "Generic file I/O error", "File not found", "File permission error", "Disk is full", "Duplicate path", "Too many files open", "System feature not enabled", "Resource file not found", "Cannot add resource", "Resource not found", "Image not found", "Image memory error", "Pen does not exist", "Config type invalid", "Config token not found", "Config parse error", "Config memory error", "Bad external code format", "Bad external code offset", "External code not present", "Null window", "Destroy window error", "Null menu", "Print aborted", "Bad print record", "Print driver error", "Windows error during printing", "Memory error during printing", "Print dialog error", "Generic print error", "Invalid device refnum", "Device not found", "Device parameter error", "Device unit error", "Cannot open device", "Device call aborted", "Generic error", "Cancelled by user", "Object ID too low", "Object ID too high", "Object not in heap", "Unknown heap", "Unknown object (invalid DefProc)", "Unknown object (DefProc not in table)", "Message out of range", "Invalid (null) method", "Unknown message", "Manager call not supported", "Bad address", "Network operation in progress", "Network operation timed out", "Connection is busy", "Network attribute not supported", "Network error", "Address in use", "System out of memory", "Connection aborted", "Connection refused", "Not connected", "Already connected", "Connection closed", "Initialization error (interapplication manager)", "Bad occurrence", "Wait on unbound occurrence handler", "Occurrence queue overflow", "Datalog type conflict", "Unused", "Unrecognized type (interapplication manager)", "Memory corrupt", "Failed to make temporary DLL", "Old CIN version", "Drag socket not found", "Failed to load drop-object", "Failed to register OLE object", "Failed to release OLE object", "Format specifier type mismatch", "Unknown format specifier", "Too few format specifiers", "Too many format specifiers", "Scan failed", "Newer CIN version", "Error converting to variant", "Runtime menu error", "Password tampered", "Variant attribute not found", "Incompatible variant data type", "Event data is not available", "Event Store is not present", "Occurrence is not found", "Event Queue is not created", "Event info is not available", "Refnum passed is NULL", "Error retrieving Class GUID", "Error retrieving CoClass GUID", "Error retrieving TypeLib GUID.", "Bad built application magic bytes.", "Specific driver is different from the specific driver associated with the Logical Name.", "There is no session opened to the class driver.", "Max Error", "MAX - Error with config objects", "MAX - Error loading configuration", "MAX - Group not supported"]
        # "Handle target error here.\nWhen this CSM try to communicate with an un-existed CSM, this CSM goes into this case."
        # "Handle mistyped state name (developer tool)"
        n50 = Format Into String(format string="Software Exception: Target \"%s\" does not exists." ("message"), error in=w169, w164) -> (resulting string=w171:string, error out=w170:errorcluster)  [unwired: 1 in]
        n51 = call <vilib>:"Error Cluster From Error Code.vi"("show call chain? (False)"=TRUE, "error in (no error)"=w170, "error message (\"\")"=w171, "error code (0)"=w172) -> ("error out"=w163:errorcluster)  [unwired: 5 in]
        n52 = call <vilib>:"Add State(s) to Queue__JKI_lib_State_Machine.vi"("State(s) in (\"\")"=w168) -> ("States Out"=w167:string)  [unwired: 14 in]
      }
      frame "Initialize Core Data" {
        # "Do not delete, rename, or modify this frame.\n(this is used to determine panel behavior on exit)"
        # "originally closed?"
        # "exe?"
        # "If panel starts closed or is an EXE, then close it when we exit"
        n53 = property class="VI"() -> ("FP.State"=w177:T4)  [unwired: 2 in, 2 out]
        n54 = property class="App"() -> ("App.Kind"=w183:T5)  [unwired: 2 in, 2 out]
        n55 = control-ref of="Current VI Reference"() -> (w178:refnum<vi>)
        n56 = Equal?(x=w177, y=T4."Closed" ("Front Panel Window:State")) -> (x = y?=w175:bool)
        n57 = Equal?(x=w183, y=T5."Run Time System" ("Application:Kind")) -> (x = y?=w181:bool)
        n58 = Or(x=w175, y=w181) -> (x .or. y?=w179:bool)
        n59 = Bundle By Name(cluster=w180, "Core.Current VI Reference"=w178, "Core.Close Panel on Exit?"=w179) -> (w185:T9)
        n60 = call <vilib>:"Add State(s) to Queue__JKI_lib_State_Machine.vi"("State(s) in (\"\")"=w187) -> ("States Out"=w186:string)  [unwired: 14 in]
      }
      frame "Async Response", "Response" {
      }
      frame "Async Message Posted" {
      }
      frame "Exit" {
        # "Do not put any code in this frame.\n(No errors that occur here will be handled.)"
        n61 = call <vilib>:"Add State(s) to Queue__JKI_lib_State_Machine.vi"("State(s) in (\"\")"=w201) -> ("States Out"=w200:string)  [unwired: 14 in]
      }
      frame "---------- Data ----------" {
        # "Do not put any code in this frame.\n(It is a separator no-op. You can make a copy of this frame to create a new Data frame)"
        n62 = call <vilib>:"Add State(s) to Queue__JKI_lib_State_Machine.vi"("State(s) in (\"\")"=w206) -> ("States Out"=w205:string)  [unwired: 14 in]
      }
      frame "Data: Initialize" {
        w207 = timestamp(0 s since 1904-01-01)  # timestamp
        w208 = 200  # Number of Samples/ch
        w214 = enum16{"Idle", "Acquiring"}."Idle"  # State
        w212 = T10 {"Device ID"=0, "SamplePeroid(ms)"=200, "Sound Format"={"sample rate (S/s)"=20000.0, "number of channels"=1, "bits per sample"=16}}  # Configuration
        w215 = T7 {"Current VI Reference"=refnum, "Close Panel on Exit?"=FALSE}  # Core
        n63 = Bundle("Core"=w215, "Configuration"=w212, "State"=w214, "Number of Samples/ch"=w208, "timestamp"=w207) -> (w216:T9)  [unwired: 1 in]
        n64 = call "CSM - Read Cluster Elements From Session.vim"("Section Name (\"\" as Default)"=w213, "Cluster"=w212) -> ("error out"=w209:errorcluster, "Cluster out"=w210:T10)  [unwired: 6 in]
        n65 = Bundle By Name(cluster=w216, "Configuration"=w210) -> (w211:T9)
        n66 = call <vilib>:"Add State(s) to Queue__JKI_lib_State_Machine.vi"("State(s) in (\"\")"=w218) -> ("States Out"=w217:string)  [unwired: 14 in]
      }
      frame "Data: Update Indicators" {
        n67 = Unbundle By Name(w221) -> ("Configuration.SamplePeroid(ms)"=w222:i32, "Configuration.Device ID"=w219:u32)
        n68 = local write "SamplePeroid(ms)"(w222) -> ()
        n69 = local write "Device ID"(w219) -> ()
      }
      frame "Data: Set Configuration" {
        n70 = call "Convert API String Arguments to Data.vim"("Reference Type"=w229, "API String"=w228) -> ("error out"=w226:errorcluster, "Data"=w227:T9)  [unwired: 6 in]
      }
      frame "Data: Get Configuration", "Data: Get Internal Data" {
        n71 = call "Query Data as API String Arguments.vim"("Name"=w234, "Cluster Data"=w236) -> ("error"=w232:errorcluster, "API String"=w233:string, "Cluster Data (dup)"=w235:T9)  [unwired: 7 in]
      }
      frame "Data: Cleanup" {
        # "Cleanup any data and references, here.\n(this is called automatically, by the Macro: Exit)"
        n72 = Unbundle By Name(w239) -> ("Core.Current VI Reference"=w242:refnum<vi>)
        n73 = Close Reference(reference=w242, error in (no error)=w241) -> (error out=w240:errorcluster)
        n74 = call <vilib>:"Add State(s) to Queue__JKI_lib_State_Machine.vi"("State(s) in (\"\")"=w244) -> ("States Out"=w243:string)  [unwired: 14 in]
      }
      frame "---------- Macro ----------" {
        # "Do not put any code in this frame.\n(It is a separator no-op. You can make a copy of this frame to create a new Macro frame)"
        n75 = call <vilib>:"Add State(s) to Queue__JKI_lib_State_Machine.vi"("State(s) in (\"\")"=w249) -> ("States Out"=w248:string)  [unwired: 14 in]
      }
      frame "Macro: Initialize" {
        n76 = call <vilib>:"Add State(s) to Queue__JKI_lib_State_Machine.vi"("State(s) in Front (\"\")"="Data: Initialize\nInitialize Core Data\nData: Update Indicators", "State(s) in (\"\")"=w255) -> ("States Out"=w254:string)  [unwired: 13 in]
      }
      frame "Macro: Exit" {
        w257 = "//Try to close device if needed\nDAQ: Close\n\nData: Cleanup\nExit"  # //Try to close device if needed DAQ: Close  Data: Cleanup Exit
        n77 = call <vilib>:"Add State(s) to Queue__JKI_lib_State_Machine.vi"("State(s) in Front (\"\")"=w257, "State(s) in (\"\")"=w261) -> ("States Out"=w260:string)  [unwired: 13 in]
      }
      frame "---------- API ----------" {
      }
      frame "API: Start" {
        # "#CSM-NOTE\nhttps://github.com/NEVSTOP-LAB/CSM-Continuous-Meausrement-and-Logging/issues/21\n\nUse CSM-Loop Support to define a loop in CSM, which is recommanded."
        n78 = Unbundle By Name(w272) -> ("State"=w273:enum16{"Idle", "Acquiring"})
        n79 = case shown="\"Acquiring\"" w273 {
          selector: w273 -> [w275 _]
          tunnel: [w275 enum16{"Idle", "Acquiring"}."Acquiring" ("Acquisition State")] -> w274
          tunnel: [_ "DAQ: Initialize \nDAQ: Configure\nDAQ: Start\nDAQ: Acquisite\nContinuous Check >> DAQ: Acquisite -><loop> \nDAQ: Stop\nDAQ: Close " ("State(s) in Front (\"\")")] -> w267
          frame "Acquiring" {
            # "The system is already acquiring. Ignore the \"Start\" message."
          }
          frame "Idle" {
            # "If the system is idle, start the acquisition."
          }
        }
        n80 = call <userlib>:"CSMLS - Define Loop State(s).vi"("Loop States"=w267, "States Queue"=w269) -> ("Remaining States"=w268:string)  [unwired: 13 in]
        n81 = Bundle By Name(cluster=w272, "State"=w274) -> (w271:T9)
      }
      frame "API: Stop" {
        # "Copy/Rename this case for your own API"
        n82 = Unbundle By Name(w279) -> ("State"=w284:enum16{"Idle", "Acquiring"})
        n83 = case shown="\"Acquiring\"" w284 {
          tunnel: ["Break Continuous" ("State(s) in Front (\"\")") _] -> w280
          frame "Acquiring" {
            # "If the system is acquiring, stop the acquisition."
          }
          frame "Idle" {
            # "The system is already idle. Ignore the \"Stop\" message."
          }
        }
        n84 = call <vilib>:"Add State(s) to Queue__JKI_lib_State_Machine.vi"("State(s) in Front (\"\")"=w280, "State(s) in (\"\")"=w283) -> ("States Out"=w282:string)  [unwired: 13 in]
      }
      frame "API: Update Settings" {
        # "#CSM-NOTE\nSync with ini-variable, to make sure the configuration could be stored in CSM INI-Variable configuration file."
        # "#CSM-NOTE\nUse this method to identify the argument type."
        n85 = Unbundle By Name(w295) -> ("Configuration"=w294:T10)
        n86 = call <userlib>:"CSM - Argument Type.vi"("Arguments"=w293) -> ("Argument Type"=w290:string, "Arguments (Dup)"=w291:string)  [unwired: 3 in]
        n87 = case shown="\"HexStr\"" w290 {
          tunnel: w294 -> [w300 w306]
          tunnel: [w299 w305] -> w287
          tunnel: [w298 w304] -> w292
          tunnel: w291 -> [w302 w303]
          frame "HexStr" {
            n88 = call <userlib>:"CSM - Convert HexStr to Data.vi"("HEX String"=w302) -> ("Variant"=w301:variant)  [unwired: 7 in, 1 out]
            n89 = Variant To Data(type=w300, Variant=w301) -> (data=w299:T10, error out=w298:errorcluster)  [unwired: 1 in]
          }
          frame Default {
            n90 = call "Convert API String Arguments to Data.vim"("Reference Type"=w306, "API String"=w303) -> ("error out"=w304:errorcluster, "Data"=w305:T10)  [unwired: 6 in]
          }
        }
        n91 = call "CSM - Write Configuration Variable.vim"("Section Name (\"\" as Default)"=w288, "error in (no error)"=w292, "Configuration"=w287) -> ("error out"=w289:errorcluster)  [unwired: 5 in, 1 out]
        n92 = Bundle By Name(cluster=w295, "Configuration"=w287) -> (w296:T9)
      }
      frame "---------- DAQ ----------" {
      }
      frame "DAQ: Initialize" {
        w321 = T11 1 items=["Finite Samples", "Continuous Samples"] ("sample mode")
        n93 = Unbundle By Name(w322) -> ("Configuration.Device ID"=w320:u32, "Configuration.SamplePeroid(ms)"=w317:i32, "Configuration.Sound Format"=w315:T8)
        n94 = Unbundle By Name(w315) -> ("sample rate (S/s)"=w314:dbl)
        n95 = Divide(x=1000, y=w317) -> (x/y=w313:dbl)
        n96 = Divide(x=w314, y=w313) -> (x/y=w311:dbl)
        n97 = Bundle By Name(cluster=w322, "Number of Samples/ch"=w311) -> (w312:T9)
        n98 = call <vilib>:"Sound Input Configure.vi"("number of samples/ch"=w311, "sample mode"=w321, "sound format"=w315, "device ID"=w320) -> ("error out"=w319:errorcluster, "task ID"=w318:T12)  [unwired: 6 in]
      }
      frame "DAQ: Configure" {
      }
      frame "DAQ: Start" {
        n99 = Get Date/Time In Seconds() -> (seconds since 1Jan1904=w327:timestamp)
        n100 = Bundle By Name(cluster=w330, "timestamp"=w327) -> (w328:T9)
      }
      frame "DAQ: Acquisite" {
        n101 = Unbundle By Name(w342) -> ("Number of Samples/ch"=w334:i32, "State"=w346:enum16{"Idle", "Acquiring"}, "timestamp"=w333:timestamp)
        n102 = case shown="\"Acquiring\"" w346 {
          tunnel: [w349 w358] -> w344
          tunnel: w345 -> [w349 w357]
          tunnel: [w348 w360] -> w343
          tunnel: w342 -> [w348 w360]
          tunnel: [_ w359] -> w338
          tunnel: w336 -> [w347 w355]
          tunnel: [w347 w354] -> w335
          tunnel: w334 -> [_ w353]
          tunnel: w333 -> [_ w350]
          frame "Idle" {
            # "Ignore \"Acquire\" messages when the acquisition is idle."
          }
          frame "Acquiring" {
            # "Acquire more data while in the \"Acquiring\" state."
            n103 = call-poly <vilib>:"Sound Input Read.vi"("number of samples/ch"=w353, "error in (no error)"=w357, "task ID"=w355) -> ("error out"=w356:errorcluster, "data"=w352:waveform(dbl)[], "task ID out"=w354:T12)  [unwired: 6 in]
            n104 = for {
              tunnel: w352 -> [w367] mode=indexing
              tunnel: [w362] -> w351 mode=indexing
              tunnel: w350 -> [w361]
              i -> [w365]
              n105 = Format Into String(format string="SoundCard_CH%d" ("name"), w365) -> (resulting string=w363:string)  [unwired: 2 in, 1 out]
              n106 = Set Waveform Attribute(5:w363, 6:"NI_ChannelName" ("name"), 7:w367) -> (3:w366:waveform(dbl))  [unwired: 1 in, 2 out]
              n107 = Bundle By Name(cluster=w366, "t0"=w361) -> (w362:waveform(dbl))
            }
            "Raw Data" <- w351
            n108 = call "CSM - Convert MassData to Argument.vim"("error in (no error)"=w356, "Data"=w351) -> ("error out"=w358:errorcluster, "MassData Argument"=w359:string)  [unwired: 6 in]
          }
        }
        n109 = call <vilib>:"Build State String with Arguments__JKI_lib_State_Machine.vi"("Arguments (\"\")"=w338, "State"="Acquired Waveform" ("Status with Arguments")) -> ("State with Arguments"=w337:string)  [unwired: 4 in]
        n110 = call <userlib>:"CSM - Broadcast Status Change.vi"("Status With Arguments"=w337, "State Queue"=w340) -> ("Remaining States"=w341:string)  [unwired: 13 in]
      }
      frame "DAQ: Stop" {
        n111 = Bundle By Name(cluster=w372, "State"=enum16{"Idle", "Acquiring"}."Idle" ("Acquisition State")) -> (w371:T9)
      }
      frame "DAQ: Close" {
        n112 = call <vilib>:"Sound Input Clear.vi"("task ID"=w376) -> ("error out"=w375:errorcluster)  [unwired: 10 in]
        n113 = call <vilib>:"Clear Errors.vi"("error in (no error)"=w375) -> ("error out"=w374:errorcluster)  [unwired: 5 in, 1 out]
      }
      frame "---------- Control Logic ----------" {
      }
      frame "Continuous Check" {
        n114 = in-place {
          n115 = in-place-cluster #1(w387) -> ("Configuration.SamplePeroid(ms)"=w392:i32, "timestamp"=w395:timestamp)
          n116 = Divide(x=w392, y=1000 ("x")) -> (x/y=w393:dbl)
          n117 = Add(x=w395, y=w393) -> (x+y=w394:timestamp)
          n118 = in-place-cluster #1("Configuration.SamplePeroid(ms)"=w392, "timestamp"=w394) -> (w383:T9)
        }
        n119 = call <userlib>:"CSMLS - Append Continuous State.vi"("Loop State(s) And Arguments"=w385, "Continous Arguments (\"\")"=w385, "Continous State"=w386, "States Queue"=w389) -> ("Remaining States"=w388:string)  [unwired: 7 in]
      }
      frame "Break Continuous" {
        n120 = call <userlib>:"CSMLS - Remove Loop Tag to Break.vi"("States Queue"=w398) -> ("Remaining States"=w397:string)  [unwired: 10 in]
      }
      frame "---------- DoSth ----------" {
      }
      frame "Do: Front Panel State" {
        n121 = Unbundle By Name(w410) -> ("Core.Current VI Reference"=w406:refnum<vi>)
        n122 = case shown="\"Hidden\", \"Hide\"" w408 {
          tunnel: w409 -> [w417 w432 w443 w456 w469]
          tunnel: [w419 w433 w445 w458 w471] -> w407
          tunnel: w406 -> [w418 w430 w444 w457 w470]
          frame "Open", "Standard", Default {
            w412 = T4."Standard" ("State")
            n123 = property class="VI"(reference=w418, error in=w417) -> (reference out=w415:refnum<vi>, error out=w416:errorcluster, "FP.State"=w414:T4)
            n124 = Not Equal?(x=w414, y=w412) -> (x != y?=w413:bool)
            n125 = case shown="True" w413 {
              tunnel: [w423 w425] -> w419
              tunnel: w416 -> [w422 w425]
              tunnel: w415 -> [w421 _]
              tunnel: w412 -> [w420 _]
              frame True {
                n126 = invoke class="VI" method="FP.Open"(reference=w421, error in=w422, "Activate"=TRUE, "State"=w420) -> (error out=w423:errorcluster)  [unwired: 1 in, 4 out]
              }
              frame False {
              }
            }
          }
          frame "Close", "Closed" {
            n127 = property class="VI"(reference=w430, error in=w432) -> (reference out=w429:refnum<vi>, error out=w431:errorcluster, "FP.State"=w427:T4)
            n128 = Not Equal?(x=w427, y=T4."Closed" ("Front Panel Window:State")) -> (x != y?=w426:bool)
            n129 = case shown="True" w426 {
              tunnel: [w434 w437] -> w433
              tunnel: w431 -> [w434 w436]
              tunnel: w429 -> [_ w435]
              frame False {
              }
              frame True {
                n130 = invoke class="VI" method="FP.Close"(reference=w435, error in=w436) -> (error out=w437:errorcluster)  [unwired: 1 in, 2 out]
              }
            }
          }
          frame "Hidden", "Hide" {
            w438 = T4."Hidden" ("State")
            n131 = property class="VI"(reference=w444, error in=w443) -> (reference out=w441:refnum<vi>, error out=w442:errorcluster, "FP.State"=w440:T4)
            n132 = Not Equal?(x=w440, y=w438) -> (x != y?=w439:bool)
            n133 = case shown="True" w439 {
              tunnel: [w449 w450] -> w445
              tunnel: w442 -> [w448 w450]
              tunnel: w441 -> [w447 _]
              tunnel: w438 -> [w446 _]
              frame True {
                n134 = invoke class="VI" method="FP.Open"(reference=w447, error in=w448, "State"=w446) -> (error out=w449:errorcluster)  [unwired: 2 in, 4 out]
              }
              frame False {
              }
            }
          }
          frame "Minimize", "Minimized" {
            w451 = T4."Minimized" ("State")
            n135 = property class="VI"(reference=w457, error in=w456) -> (reference out=w454:refnum<vi>, error out=w455:errorcluster, "FP.State"=w453:T4)
            n136 = Not Equal?(x=w453, y=w451) -> (x != y?=w452:bool)
            n137 = case shown="True" w452 {
              tunnel: [w462 w463] -> w458
              tunnel: w455 -> [w461 w463]
              tunnel: w454 -> [w460 _]
              tunnel: w451 -> [w459 _]
              frame True {
                n138 = invoke class="VI" method="FP.Open"(reference=w460, error in=w461, "State"=w459) -> (error out=w462:errorcluster)  [unwired: 2 in, 4 out]
              }
              frame False {
              }
            }
          }
          frame "Maximize", "Maximized" {
            w464 = T4."Maximized" ("State")
            n139 = property class="VI"(reference=w470, error in=w469) -> (reference out=w467:refnum<vi>, error out=w468:errorcluster, "FP.State"=w466:T4)
            n140 = Not Equal?(x=w466, y=w464) -> (x != y?=w465:bool)
            n141 = case shown="True" w465 {
              tunnel: [w475 w476] -> w471
              tunnel: w468 -> [w474 w476]
              tunnel: w467 -> [w473 _]
              tunnel: w464 -> [w472 _]
              frame True {
                n142 = invoke class="VI" method="FP.Open"(reference=w473, error in=w474, "State"=w472) -> (error out=w475:errorcluster)  [unwired: 2 in, 4 out]
              }
              frame False {
              }
            }
          }
        }
      }
      frame "Do: Hide FP and Exit When stand-alone" {
        # "#CSM-NOTE\nNo parent"
        n143 = Call Chain() -> (call chain=w480:string[])
        n144 = Array Size(array=w480) -> (size(s)=w479:i32)
        n145 = Equal?(x=1, y=w479) -> (x = y?=w477:bool)
        n146 = call-poly <userlib>:"Add State(s) to Queue By BOOL++.vi"("TRUE (\"\")"="Macro: Exit" ("State(s) at Back (\"\")"), "Condition"=w477, "State Queue (\"\")"="Do: Front Panel State >> Hide" ("State(s) at Back (\"\")")) -> ("Remaining States"=w481:string)  [unwired: 8 in]
        n147 = call <vilib>:"Add State(s) to Queue__JKI_lib_State_Machine.vi"("State(s) in Front (\"\")"=w481, "State(s) in (\"\")"=w482) -> ("States Out"=w483:string)  [unwired: 13 in]
      }
    }
  }
